vi "QR_readerV2.vi"() -> ()   [LabVIEW 2017]
uses:
  GlobalVariable.vi
  <vilib>/vision/NI_Vision_Development_Module.lvlib
panel:
  out "only_cube":u8[](array[numeric])
  out "array_alpha":u8[](array[numeric])
  out "appended array":string[](array[string])
  out "alpha_only":u8[](array[numeric])
  out "QR_array":string[](array[string])
  in  "Stop (F)":bool
  out "Barcode Data":string
  out "Image Display":T1(plugin-control)
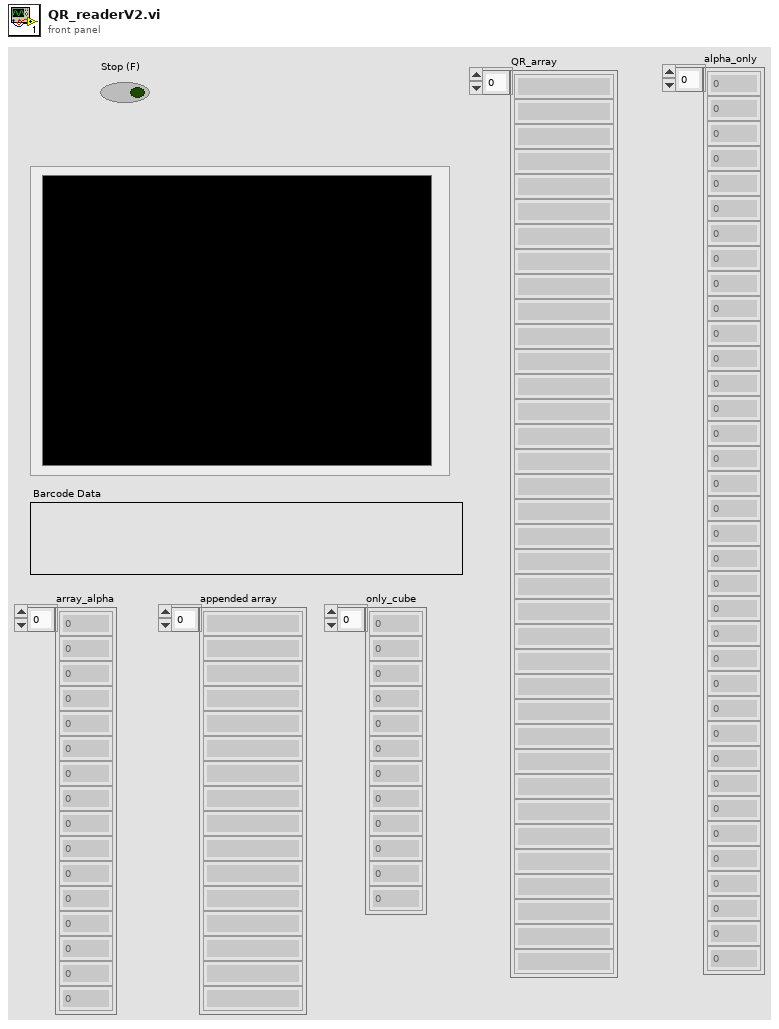
[diagram p1: front panel]
types:
  T1 = typedef "IMAQ Image.ctl" = refnum<image>
  T2 = typedef "QR Code Report.ctl" = cluster{"Found?":bool, "Data":string, "Bounding Box":cluster{"x":sgl, "y":sgl}[], "Errors Corrected":u32, "Dimensions (Rows/Cols)":u32, "Version":u32, "QR Model":T3, "Stream Mode":T4, "Barcode Polarity":T5, "Mirrored?":bool, "Append Stream Position":u32, "Size of Append Stream":u32, "First EAN-128 ID":i32, "First Alternate Language ID":i32, "Append Stream ID":u32, "Minimum Edge Strength":u32, "Demodulation Mode":T6, "Cell Sample Size":T7, "Cell Filter Mode":T8}
  T3 = typedef "QR Code Model Type.ctl" = i32
  T4 = typedef "QR Code Stream Mode Type.ctl" = i32
  T5 = typedef "Data Matrix Polarity.ctl" = i32
  T6 = typedef "Demodulation Mode.ctl" = i32
  T7 = typedef "Cell Sample Size.ctl" = i32
  T8 = typedef "Cell Filter Mode.ctl" = i32
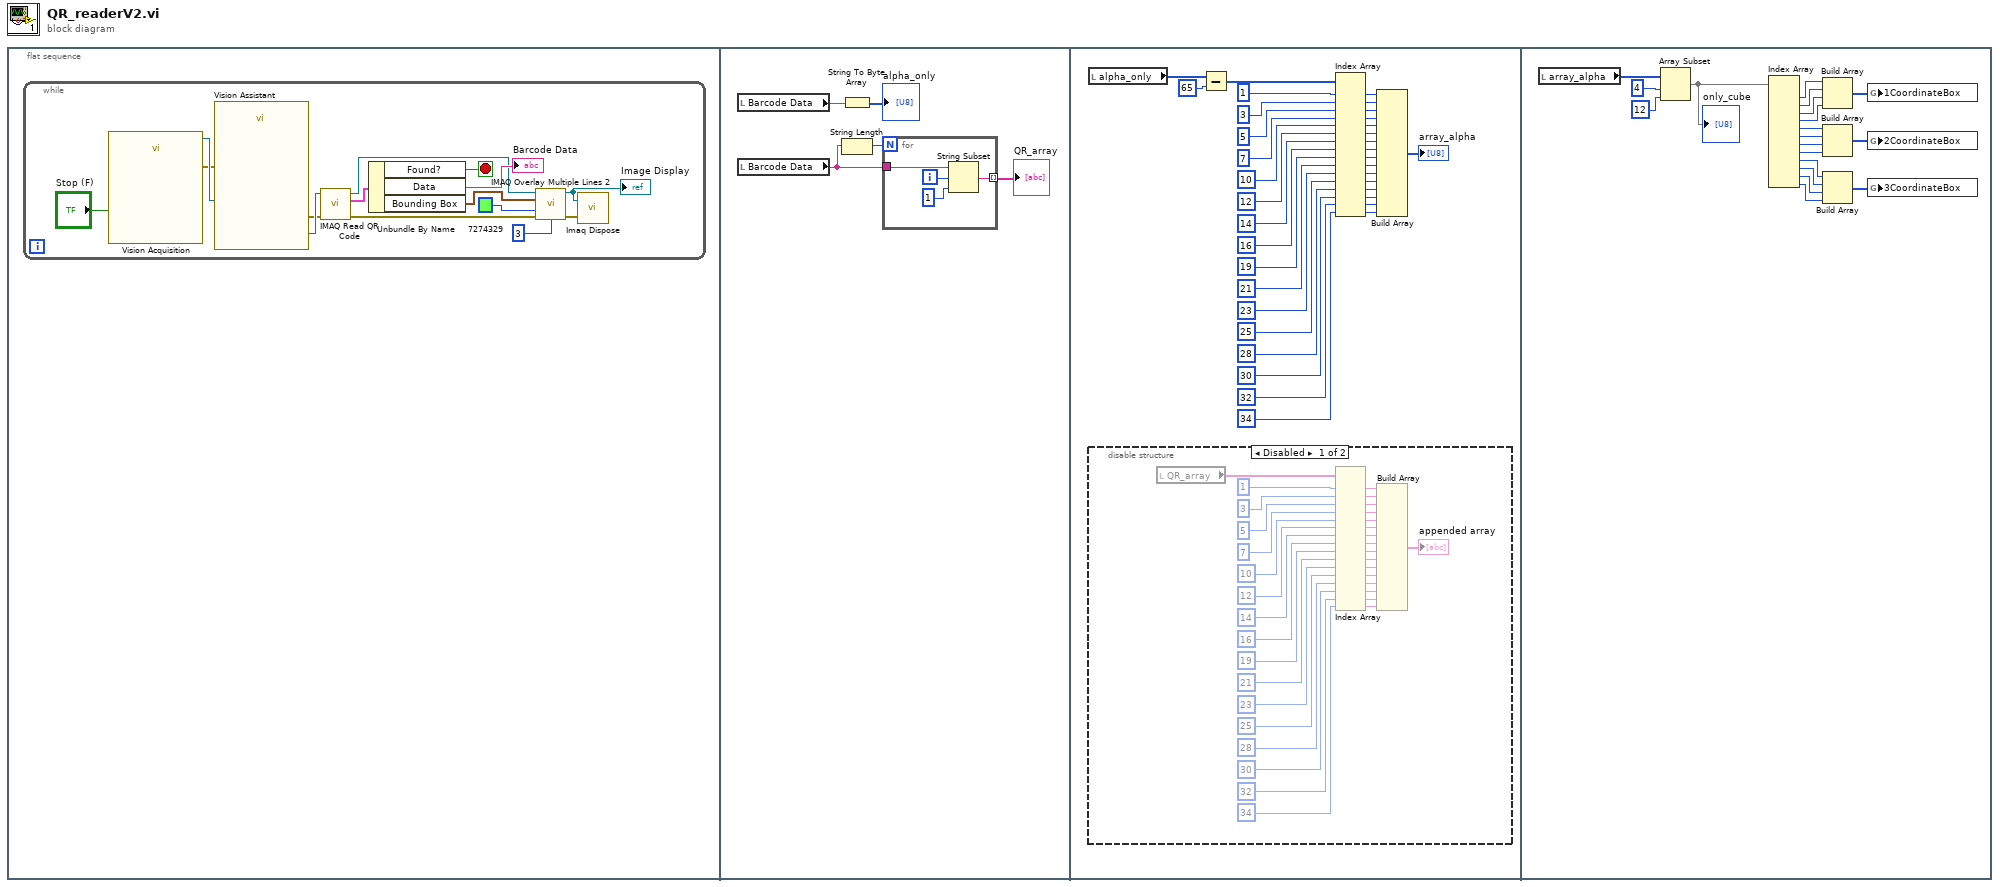
[diagram p0: block diagram]
diagram:
  n1 = flat-sequence {
    frame #0 {
      n2 = while {
        stop <- w8 stop-if-true
        n3 = call "Vision Acquisition"("Stop (F)"="Stop (F)") -> ("Image Out"=w13:T1, "error out"=w10:errorcluster)  [unwired: 24 in, 1 out]
        n4 = call "Vision Assistant"("Image In"=w13, "error in"=w10) -> ("Image Out"=w12:T1, "error out"=w11:errorcluster)  [unwired: 24 in]
        n5 = call "IMAQ Read QR Code"("error in (no error)"=w11, "Image"=w12) -> ("error out"=w2:errorcluster, "QR Code Report"=w14:T2, "Image (duplicate)"=w1:T1)  [unwired: 6 in, 1 out]
        n6 = Unbundle By Name(w14) -> ("Found?"=w8:bool, "Data"=→"Barcode Data":string, "Bounding Box"=w3:cluster{"x":sgl, "y":sgl}[])
        n7 = call "IMAQ Overlay Multiple Lines 2"("Image"=w1, "Line End Points"=w3, "Color"=u32 7274329, "error in (no error)"=w2, "Width"=u32 3) -> ("Image Out"=w7:T1, "error out"=w6:errorcluster)  [unwired: 9 in]
        "Image Display" <- w7
        n8 = call "Imaq Dispose"("Image"=w7, "error in (no error)"=w6) -> ()  [unwired: 4 in, 1 out]
      }
    }
    frame #1 {
      n9 = local read "Barcode Data"() -> (w16:string)
      n10 = local read "Barcode Data"() -> (w19:string)
      n11 = String To Byte Array(string=w16) -> (unsigned byte array=→"alpha_only":u8[])
      n12 = String Length(string=w19) -> (length=w20:i32)
      n13 = for {
        N: w20 -> [_]
        tunnel: [w24] -> w18 mode=indexing
        tunnel: w19 -> [w21]
        i -> [w22]
        n14 = String Subset(string=w21, offset (0)=w22, length (rest)=1 ("length (rest)")) -> (substring=w24:string)
      }
      "QR_array" <- w18
    }
    frame #2 {
      n15 = local read "alpha_only"() -> (w27:u8[])
      n16 = disable-structure shown="Disabled" {
        frame Disabled {
          n17 = local read "QR_array"() -> (w78:string[])
          n18 = Index Array(array=w78, index #1=1 ("index"), index #2=3 ("index"), index #3=5 ("index"), index #4=7 ("index"), index #5=10 ("index"), index #6=12 ("index"), index #7=14 ("index"), index #8=16 ("index"), index #9=19 ("index"), index #10=21 ("index"), index #11=23 ("index"), index #12=25 ("index"), index #13=28 ("index"), index #14=30 ("index"), index #15=32 ("index"), index #16=34 ("index")) -> (element #1=w77:string, element #2=w76:string, element #3=w75:string, element #4=w74:string, element #5=w72:string, element #6=w73:string, element #7=w71:string, element #8=w70:string, element #9=w69:string, element #10=w68:string, element #11=w67:string, element #12=w66:string, element #13=w65:string, element #14=w64:string, element #15=w63:string, element #16=w62:string)
          n19 = Build Array(w77, w76, w75, w74, w72, w73, w71, w70, w69, w68, w67, w66, w65, w64, w63, w62) -> (→"appended array":string[])
        }
        frame Enabled {
        }
      }
      n20 = Subtract(x=w27, y=65) -> (x-y=w26:i32[])
      n21 = Index Array(array=w26, index #1=1 ("index"), index #2=3 ("index"), index #3=5 ("index"), index #4=7 ("index"), index #5=10 ("index"), index #6=12 ("index"), index #7=14 ("index"), index #8=16 ("index"), index #9=19 ("index"), index #10=21 ("index"), index #11=23 ("index"), index #12=25 ("index"), index #13=28 ("index"), index #14=30 ("index"), index #15=32 ("index"), index #16=34 ("index")) -> (element #1=w44:i32, element #2=w43:i32, element #3=w42:i32, element #4=w41:i32, element #5=w39:i32, element #6=w40:i32, element #7=w38:i32, element #8=w37:i32, element #9=w36:i32, element #10=w35:i32, element #11=w34:i32, element #12=w33:i32, element #13=w32:i32, element #14=w31:i32, element #15=w30:i32, element #16=w29:i32)
      n22 = Build Array(w44, w43, w42, w41, w39, w40, w38, w37, w36, w35, w34, w33, w32, w31, w30, w29) -> (→"array_alpha":i32[])
    }
    frame #3 {
      n23 = local read "array_alpha"() -> (w113:u8[])
      n24 = Array Subset(array=w113, index=4, length=12) -> (w110:u8[])
      "only_cube" <- w110
      n25 = Index Array(array=w110) -> (element #1=w109:u8, element #2=w108:u8, element #3=w107:u8, element #4=w106:u8, element #5=w104:u8, element #6=w103:u8, element #7=w102:u8, element #8=w101:u8, element #9=w99:u8, element #10=w98:u8, element #11=w97:u8, element #12=w96:u8)  [unwired: 12 in]
      n26 = Build Array(w109, w108, w107, w106) -> (w105:u8[])
      n27 = Build Array(w104, w103, w102, w101) -> (w100:u8[])
      n28 = Build Array(w99, w98, w97, w96) -> (w95:u8[])
      n29 = global write "GlobalVariable.vi" "1CoordinateBox"(w105) -> ()
      n30 = global write "GlobalVariable.vi" "2CoordinateBox"(w100) -> ()
      n31 = global write "GlobalVariable.vi" "3CoordinateBox"(w95) -> ()
    }
  }
